vi "Get Channels.vi"(8 "error in":errorcluster, 11 "Instrument":string="DMM") -> (0 "error out":errorcluster, 3 "Channels":T1[](array[typedef]))   [LabVIEW 2021]
uses:
  Controls/Channels.ctl
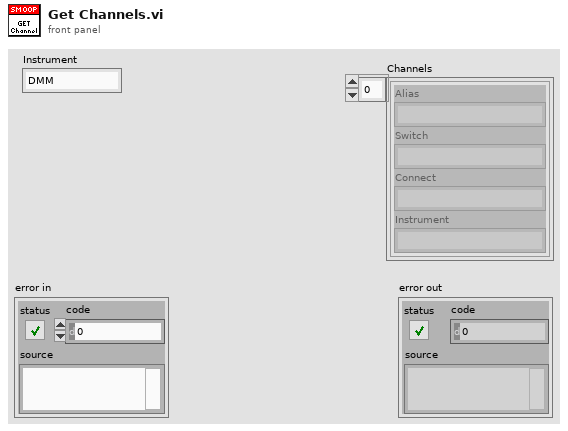
[diagram p1: front panel]
types:
  T1 = typedef "Channels.ctl" = cluster{"Alias":string, "Switch":string, "Connect":string, "Instrument":string}
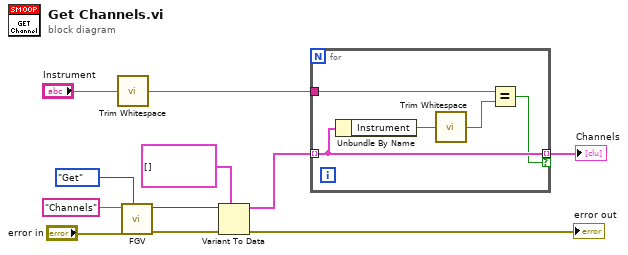
[diagram p0: block diagram]
diagram:
  n1 = call <vilib>:"Trim Whitespace.vi"("string"="Instrument") -> ("trimmed string"=w3:string)  [unwired: 1 in]
  n2 = call "FGV.vi"("Method (Get)"=enum16{"Get", "Set"}."Get", "error in"="error in", "Name"="Channels") -> ("error out"=w8:errorcluster, "Data out"=w9:variant)  [unwired: 7 in]
  n3 = Variant To Data(error in=w8, type=T1[] [], Variant=w9) -> (data=w5:T1[], error out=→"error out":errorcluster)
  n4 = for {
    tunnel: w5 -> [w13] mode=indexing
    tunnel: w3 -> [w14]
    tunnel: [w13] -> w1 mode=indexing if=w12
    n5 = Unbundle By Name(w13) -> ("Instrument"=w15:string)
    n6 = call <vilib>:"Trim Whitespace.vi"("string"=w15) -> ("trimmed string"=w16:string)  [unwired: 1 in]
    n7 = Equal?(x=w14, y=w16) -> (x = y?=w12:bool)
  }
  "Channels" <- w1
